vi "Read CB illuminance reached.vi"(8 "error in (no error)":errorcluster, 11 "Ambient Light Bricklet in":refnum<class "Ambient Light Bricklet.lvclass">) -> (0 "error out":errorcluster, 2 "CB illuminance reached":refnum<user-event>, 3 "Ambient Light Bricklet out":refnum<class "Ambient Light Bricklet.lvclass">)   [LabVIEW 2011, in "Tinkerforge.lvlib" / "Ambient Light Bricklet.lvclass"]
uses:
  Ambient Light Bricklet.lvclass
  Ambient Light Bricklet.lvclass/Ambient Light Bricklet.ctl
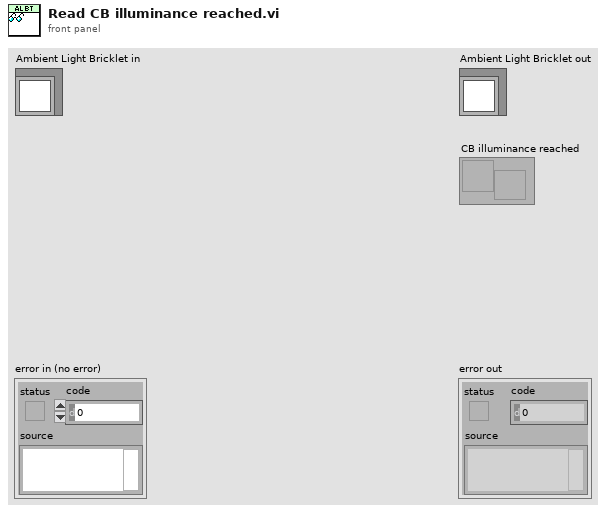
[diagram p1: front panel]
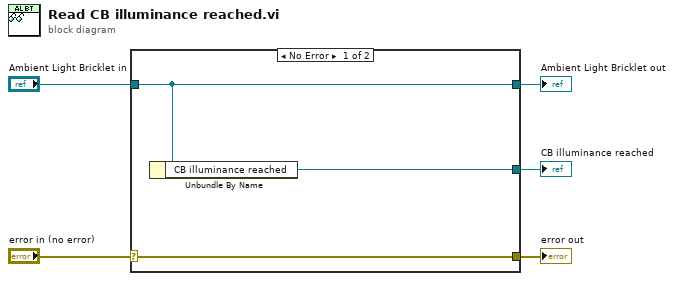
[diagram p0: block diagram]
diagram:
  n1 = case shown="No Error" "error in (no error)" {
    selector: "error in (no error)" -> [w8 w9]
    tunnel: [w8 w9] -> w4
    tunnel: [w7 w10] -> w2
    tunnel: "Ambient Light Bricklet in" -> [w7 w10]
    tunnel: [w6 _] -> w1
    frame No Error {
      n2 = Unbundle By Name(w7) -> ("CB illuminance reached"=w6:refnum<user-event>)
    }
    frame Error {
    }
  }
  "error out" <- w4
  "Ambient Light Bricklet out" <- w2
  "CB illuminance reached" <- w1
